vi "DEMO_sourcode.vi"() -> ()   [LabVIEW 2022 SP3]
panel:
  out "error out":errorcluster
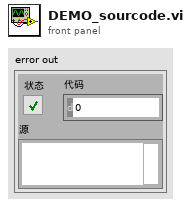
[diagram p1: front panel]
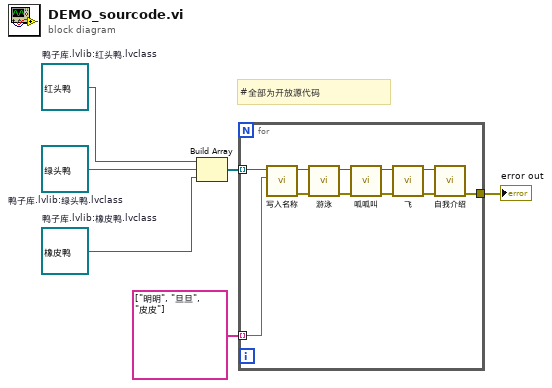
[diagram p0: block diagram]
diagram:
  w3 = refnum<class "橡皮鸭.lvclass"> refnum  # 鸭子库.lvlib:橡皮鸭.lvclass
  w4 = refnum<class "绿头鸭.lvclass"> refnum  # 鸭子库.lvlib:绿头鸭.lvclass
  w1 = refnum<class "红头鸭.lvclass"> refnum  # 鸭子库.lvlib:红头鸭.lvclass
  # "#全部为开放源代码"
  n1 = Build Array(w1, w4, w3) -> (w2:refnum<class "鸭子.lvclass">[])
  n2 = for {
    tunnel: string[] ["明明", "旦旦", "皮皮"] -> [w9] mode=indexing
    tunnel: [w8] -> w6
    tunnel: w2 -> [w7] mode=indexing
    n3 = call "写入名称.vi"("名称"=w9, "鸭子输入"=w7) -> ("error out"=w10:errorcluster, "鸭子输出"=w11:refnum<class "鸭子.lvclass">)  [unwired: 8 in]
    n4 = call-dynamic "游泳.vi"("error in (no error)"=w10, "鸭子 输入"=w11) -> ("error out"=w12:errorcluster, "鸭子 输出"=w13:refnum<class "鸭子.lvclass">)  [unwired: 8 in]
    n5 = call-dynamic "呱呱叫.vi"("error in (no error)"=w12, "鸭子 输入"=w13) -> ("error out"=w16:errorcluster, "鸭子 输出"=w14:refnum<class "鸭子.lvclass">)  [unwired: 8 in]
    n6 = call-dynamic "飞.vi"("error in (no error)"=w16, "鸭子 输入"=w14) -> ("error out"=w17:errorcluster, "鸭子 输出"=w15:refnum<class "鸭子.lvclass">)  [unwired: 8 in]
    n7 = call-dynamic "自我介绍.vi"("error in (no error)"=w17, "鸭子 输入"=w15) -> ("error out"=w8:errorcluster)  [unwired: 8 in, 1 out]
  }
  "error out" <- w6
